vi "Configure Alarm Reset Options.vi"(8 "error in (no error)":errorcluster, 9 "Alarm Reset (All Enabled)":T1={"Keyboard/Micro-Switch"=TRUE, "External"=TRUE, "Reset Parameter"=TRUE, "Automatic"=TRUE}, 10 "Node (3)":u8=3 caption="Node" min=3 max=128 step=1, 11 "VISA resource name":refnum<visa-resource-name>) -> (0 "error out":errorcluster, 3 "VISA resource name out":refnum<visa-resource-name>)   [LabVIEW 2024, in "Bronkhorst FLOW-BUS.lvlib"]
doc: "Enables control of resetting the alarm for the selected buttons/values. External is not used in MBC2 and MBC3 type instruments."
uses:
  Bronkhorst FLOW-BUS.lvlib
  Private/FLOW-BUS RW.ctl
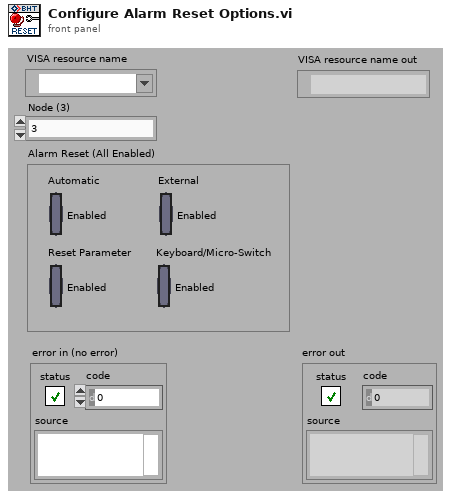
[diagram p1: front panel]
types:
  T1 = cluster{"Keyboard/Micro-Switch":bool, "External":bool, "Reset Parameter":bool, "Automatic":bool}
  T2 = typedef "Bronkhorst FLOW-BUS.lvlib/FLOW-BUS RW.ctl" = cluster{"Node Address (3)":u8, "Communication Command":enum16{"Status message", "Send parameter with destination address and 00 response", "Send parameter with destination address", "Request parameter"}, "Process (0)":u16, "Parameter (0)":u16, "Data Type (0: Character)":enum16{"Character", "Integer", "Float or Long", "String"}, "Data for Char or Int (0)":u32, "Data for Float or Long (0)":sgl, "Data for String":string, "Length of Requested String (0)":u8}
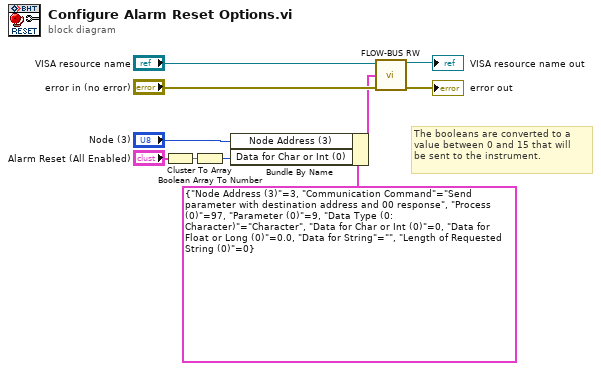
[diagram p0: block diagram]
diagram:
  # "The booleans are converted to a \nvalue between 0 and 15 that will \nbe sent to the instrument."
  n1 = Cluster To Array(cluster="Alarm Reset (All Enabled)") -> (array=w9:bool[])
  n2 = Boolean Array To Number(Boolean array=w9) -> (number=w3:u32)
  n3 = Bundle By Name(cluster=T2 {"Node Address (3)"=3, "Communication Command"=enum."Send parameter with destination address and 00 response", "Process (0)"=97, "Parameter (0)"=9, "Data Type (0: Character)"=enum."Character", "Data for Char or Int (0)"=0, "Data for Float or Long (0)"=0.0, "Data for String"="", "Length of Requested String (0)"=0} ("FLOW-BUS Command Settings"), "Node Address (3)"="Node (3)", "Data for Char or Int (0)"=w3) -> (w2:T2)
  n4 = call "FLOW-BUS RW.vi"("VISA resource name"="VISA resource name", "FLOW-BUS Command Settings"=w2, "error in (no error)"="error in (no error)") -> ("VISA resource name out"=→"VISA resource name out":refnum<visa-resource-name>, "error out"=→"error out":errorcluster)  [unwired: 8 in, 3 out]
